vi "MPU6050.vi"() -> ()   [LabVIEW 2020]
uses:
  <vilib>/MakerHub/LINX/Public/Sensors/Accelerometer/MPU60X0/DeviceAddresses.ctl
  <vilib>/MakerHub/LINX/Public/Utilities/Open Serial.vi
  <vilib>/MakerHub/LINX/LMH-LINX.lvlib
  <vilib>/MakerHub/LINX/Public/Sensors/Accelerometer/MPU60X0/MPU60X0.lvlib
panel:
  out "Waveform Chart":T1(graph)
  in  "stop":bool
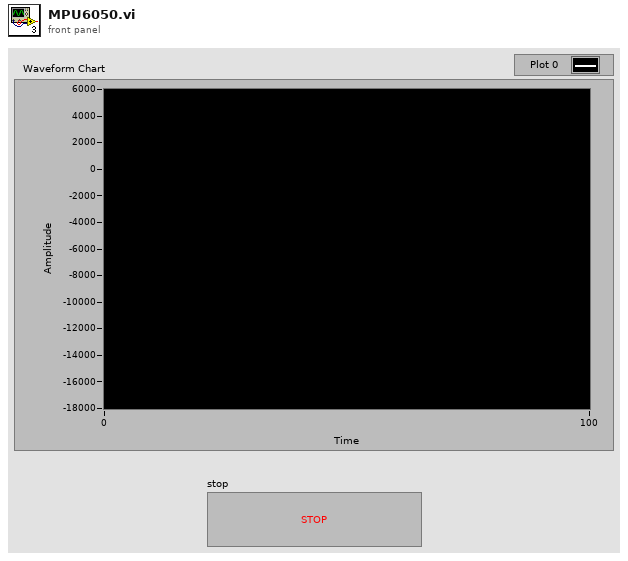
[diagram p1: front panel]
types:
  T1 = cluster{"X Axis":i16, "Y Axis":i16, "Z Axis":i16}
  T2 = typedef "LMH-LINX.lvlib/MPU60X0.lvlib/DeviceAddresses.ctl" = enum16{"0x68", "0x69"}
  T3 = typedef "LMH-LINX.lvlib/LINX Ref.ctl" = cluster{"IO":T4, "Interface":T5, "LINX Device Config":T6}
  T4 = typedef "LMH-LINX.lvlib/Platform.ctl" = enum16{"Remote", "Local"}
  T5 = typedef "LMH-LINX.lvlib/Interface.ctl" = enum16{"Serial", "TCP"}
  T6 = typedef "LMH-LINX.lvlib/Device.lvlib/LINX Device Config.ctl" = cluster{"Interface":T5, "COM Port":refnum<visa-resource-name>, "TCP Configuration":T7, "Device Family":u8, "Device ID":u8, "Device Name":string, "TCP Ref":refnum<k5>, "Channels":T8}
  T7 = typedef "LMH-LINX.lvlib/Device.lvlib/TCP Config.ctl" = cluster{"IP Address":string, "Port":u16}
  T8 = typedef "LMH-LINX.lvlib/Channels.ctl" = cluster{"DI":u8[], "DO":u8[], "AI":u8[], "AO":u8[], "PWM":u8[], "QE":u8[], "UART":u8[], "I2C 2":u8[], "SPI":u8[], "CAN":u8[], "Servo":u8[], "AI Ref (V)":dbl, "AI Resolution (Bits)":u8, "AO Ref (V)":dbl, "AO Resolution (Bits)":u8}
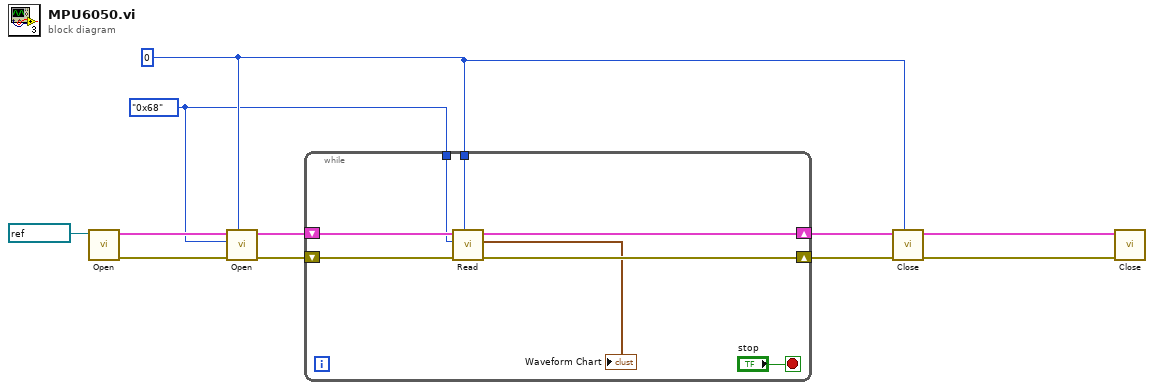
[diagram p0: block diagram]
diagram:
  w1 = DeviceAddresses."0x68" ("I2C Slave Address")
  w2 = u8 0 ("I2C Channel")
  n1 = call-poly <vilib>:"Open.vi"("Serial Port"=refnum<visa-resource-name> "COM4") -> ("Error Out"=w9:errorcluster, "LINX Resource"=w10:T3)  [unwired: 8 in, 1 out]
  n2 = call <vilib>:"Open.vi"("I2C Channel"=w2, "Error In"=w9, "I2C Slave Address"=w1, "LINX Resource"=w10) -> ("Error Out"=w7:errorcluster, "LINX Resource"=w8:T3)  [unwired: 6 in]
  n3 = while {
    tunnel: w2 -> [w15]
    tunnel: w1 -> [w14]
    shift-right: [w17] -> w6
    shift-left: w8 -> [w19]
    shift-right: [w16] -> w5
    shift-left: w7 -> [w18]
    stop <- "stop" stop-if-true
    n4 = call <vilib>:"Read.vi"("I2C Channel"=w15, "Error In"=w18, "I2C Slave Address"=w14, "LINX Resource"=w19) -> ("Error Out"=w16:errorcluster, "Acceleration Data (g)"=→"Waveform Chart":T1, "LINX Resource"=w17:T3)  [unwired: 3 in, 2 out]
  }
  n5 = call <vilib>:"Close.vi"("I2C Channel (0)"=w2, "Error In"=w5, "LINX Resource"=w6) -> ("Error Out"=w3:errorcluster, "LINX Resource"=w4:T3)  [unwired: 7 in]
  n6 = call <vilib>:"Close.vi"("Error In"=w3, "LINX Resource"=w4) -> ()  [unwired: 9 in, 1 out]
